vi "I32ArrayMsgProbe.vi"(11 "Message":refnum<class "I32ArrayMsg.lvclass">) -> (2 "Value String":string, 3 "Boolean":bool)   [LabVIEW 2018, in "LapDog.Messaging.v3.NativeArrays.lvlib" / "I32ArrayMsg.lvclass"]
uses:
  I32ArrayMsg.lvclass
  T:/git/LapDog.Messaging/src/LapDog.Messaging/Message/Message.lvclass
  LapDog.Messaging/Message/Message.lvclass
panel:
  out "Values":i32[](array[numeric])
  out "Message Type":string
  out "Array Size":string
  out "Message Name":string
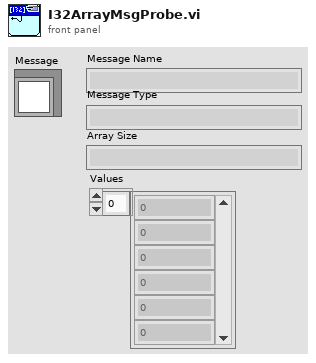
[diagram p1: front panel]
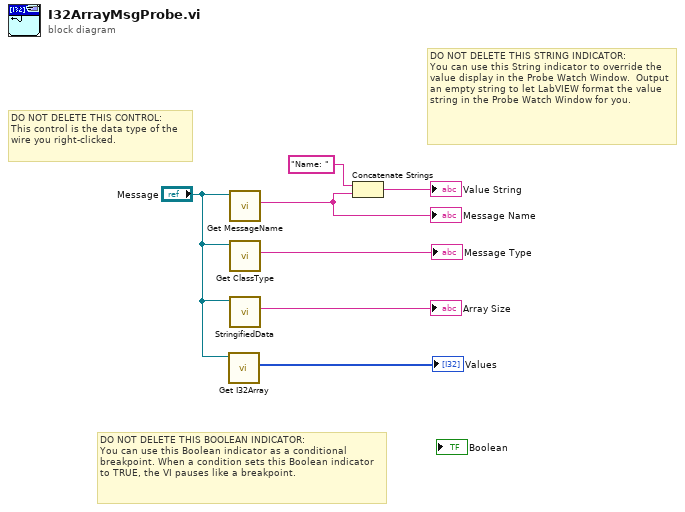
[diagram p0: block diagram]
diagram:
  # "DO NOT DELETE THIS STRING INDICATOR: \nYou can use this String indicator to override the value display in the Probe Watch Window.  Output an empty string to let LabVIEW format the value string in the Probe Watch Window for you."
  # "DO NOT DELETE THIS BOOLEAN INDICATOR: \nYou can use this Boolean indicator as a conditional breakpoint. When a condition sets this Boolean indicator to TRUE, the VI pauses like a breakpoint."
  # "DO NOT DELETE THIS CONTROL: \nThis control is the data type of the wire you right-clicked."
  n1 = call-dynamic "Get I32Array.vi"("I32ArrayMsg in"="Message") -> ("Message Data"=→"Values":i32[])  [unwired: 8 in, 2 out]
  n2 = call "Get MessageName.vi"("Message in"="Message") -> ("Message Name"=w3:string)  [unwired: 8 in, 2 out]
  "Message Name" <- w3
  n3 = call-dynamic "Get ClassType.vi"("Message in"="Message") -> ("Class Type"=→"Message Type":string)  [unwired: 8 in, 2 out]
  n4 = call-dynamic "StringifiedData.vi"("I32ArrayMsg in"="Message") -> ("Stringified Data"=→"Array Size":string)  [unwired: 8 in, 2 out]
  n5 = Concatenate Strings("Name: " ("string"), w3) -> (→"Value String":string)
